vi "iWorx - Force.vi"() -> ()   [LabVIEW 2012]
uses:
  <vilib>/DAQmx/create/channels.llb/DAQmx Create Channel (AI-Voltage-Basic).vi
  <vilib>/DAQmx/read.llb/DAQmx Read (Analog 1D Wfm NChan 1Samp).vi
  <vilib>/ptbypt/NI_PtbyPt.lvlib
panel:
  in  "Set Up":bool
  out "Offset":dbl=-0.0016949152542372892
  out "Slope":dbl=0.33898305084745767
  in  "Set SP2":bool
  in  "Set SP1":bool
  in  "Channel":u16(ring) items=["Channel 1", "Channel 2"]
  in  "Calibration Data":T1={"SP1 Voltage"=0.3, "SP2 Voltage"=0.005, "SP1 Value"=0.1, "SP2 Value"=0.0} {"SP2 Value" format="%_3f Kg"; "SP1 Value" format="%_3f Kg"; "SP2 Voltage" format="%.3f V"; "SP1 Voltage" format="%.3f V"}
  in  "Pause Button":bool
  in  "Snapshot":bool
  out "Processed Signal":dbl(knob) caption="Force (Kg)" scale=-5.0..5.0
  in  "stop":bool
  out "Waveform Chart":dbl(graph)
  in  "Sample Timing":u16(ring)=50 items=["20Hz"=50, "5 Hz"=200, "2 Hz"=500, "1 Hz"=1000, ".5 Hz"=2000, ".2 Hz"=5000]
  in  "Clear Chart":bool
  in  "Open Log":bool
  in  "Autoscale Y":bool
  out "Raw Signal":dbl(knob) scale=-2.5..2.5
  # "iWorx - Force - Data Logger"
  # "Sensor Input"
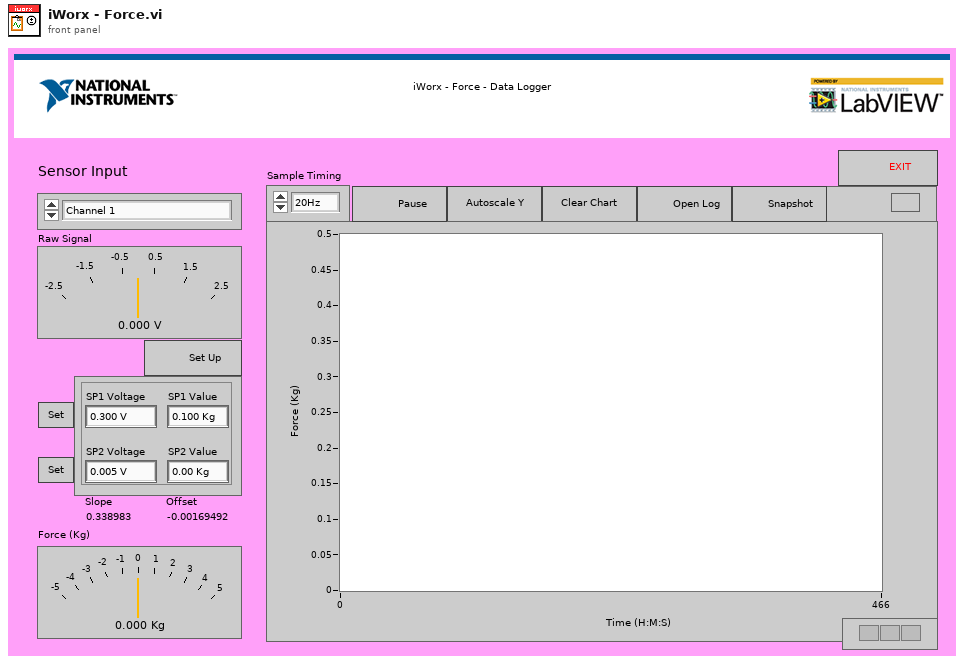
[diagram p1: front panel]
types:
  T1 = cluster{"SP1 Voltage":dbl, "SP2 Voltage":dbl, "SP1 Value":dbl, "SP2 Value":dbl}
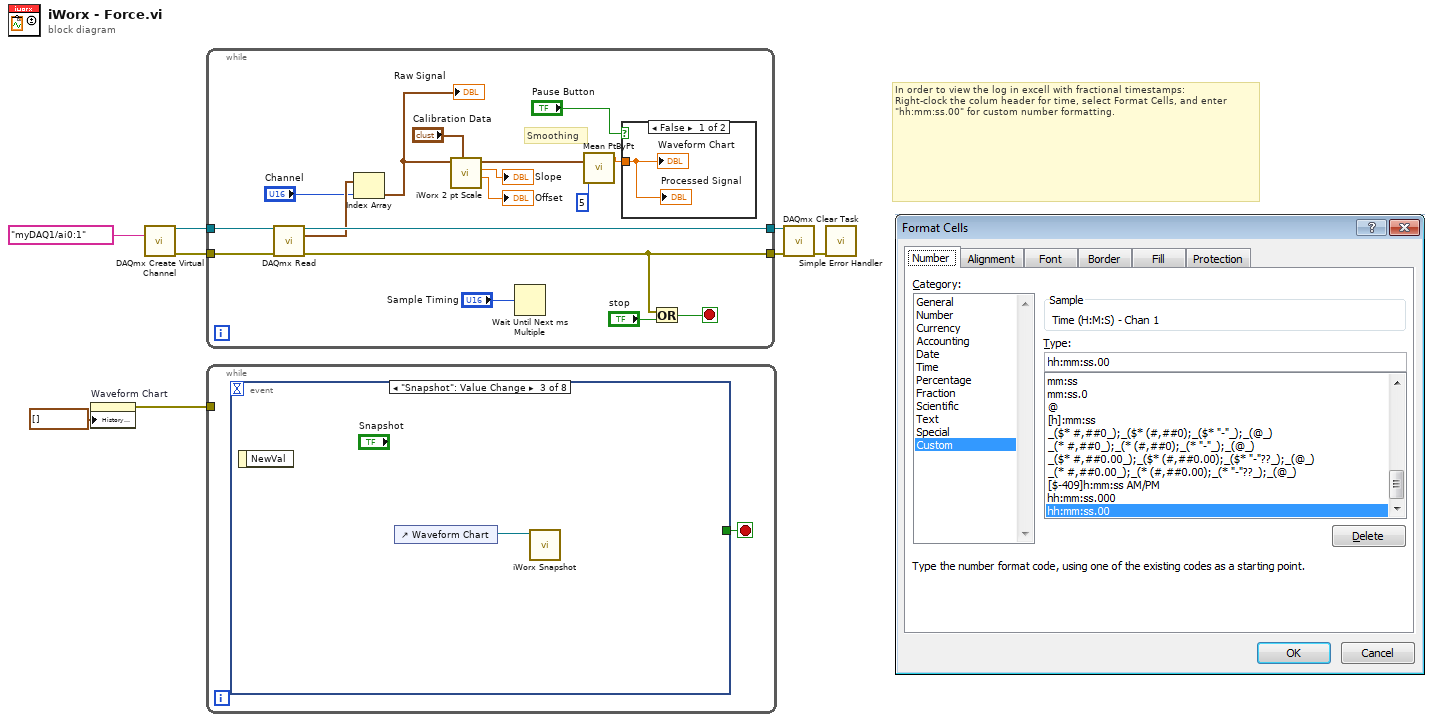
[diagram p0: block diagram]
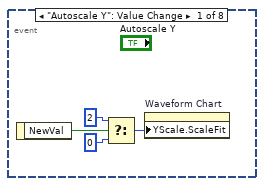
[diagram p2: hidden frame]
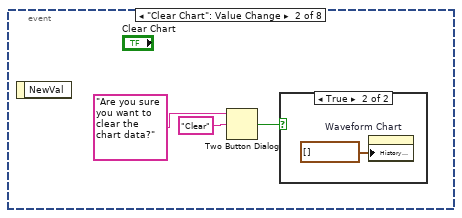
[diagram p3: hidden frame]
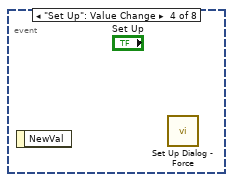
[diagram p5: hidden frame]
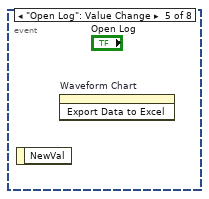
[diagram p6: hidden frame]
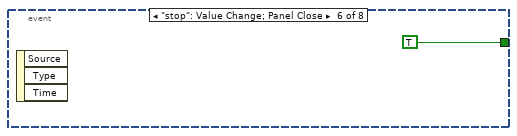
[diagram p7: hidden frame]
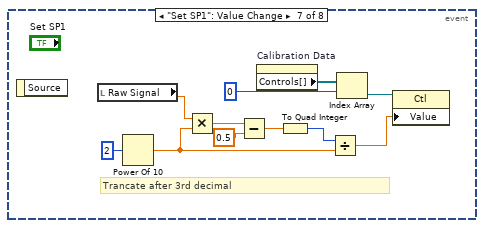
[diagram p8: hidden frame]
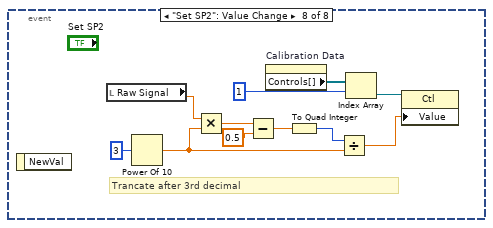
[diagram p9: hidden frame]
diagram:
  # "In order to view the log in excell with fractional timestamps: \nRight-clock the colum header for time, select Format Cells, and enter \"hh:mm:ss.00\" for custom number formatting."
  n1 = property on="Waveform Chart" class="WFChart (strict)"("History Data"=waveform(dbl)[] []) -> (error out=w3:errorcluster)  [unwired: 2 in, 1 out]
  n2 = call-poly <vilib>:"DAQmx Create Virtual Channel.vi"("physical channels"=tag "myDAQ1/ai0:1") -> ("task out"=w5:refnum<k21>, "error out"=w4:errorcluster)  [unwired: 13 in]
  n3 = while {
    tunnel: w5 -> [w23]
    tunnel: [w22] -> w8
    tunnel: w4 -> [w21]
    tunnel: [w19] -> w7
    stop <- w20 stop-if-true
    # "Smoothing"
    n4 = call-poly <vilib>:"DAQmx Read.vi"("task/channels in"=w23, "error in"=w21) -> ("task out"=w22:refnum<k21>, "data"=w17:waveform(dbl)[], "error out"=w19:errorcluster)  [unwired: 11 in]
    n5 = Index Array(array=w17, index="Channel") -> (element=w12:waveform(dbl))
    "Raw Signal" <- w12
    n6 = call "iWorx 2 pt Scale.vi"("Set Points"="Calibration Data", "Raw Waveform"=w12) -> ("Offset"=→"Offset":dbl, "Slope"=→"Slope":dbl, "Scaled Value"=w11:waveform(dbl))  [unwired: 7 in]
    n7 = Wait Until Next ms Multiple(millisecond multiple="Sample Timing") -> ()  [unwired: 1 out]
    n8 = call <vilib>:"Mean PtByPt.vi"("x"=w11, "sample length"=5) -> ("mean"=w10:dbl)  [unwired: 2 in, 1 out]
    n9 = case shown="False" "Pause Button" {
      tunnel: w10 -> [w26 _]
      frame False {
        "Waveform Chart" <- w26
        "Processed Signal" <- w26
      }
      frame True {
      }
    }
    n10 = Or(x=w19, y="stop") -> (x .or. y?=w20:bool)
  }
  n11 = while {
    tunnel: w3 -> [_]
    stop <- w27 stop-if-true
    n12 = event shown="[2] \"Snapshot\": Value Change" {
      selector: _ -> [_ _ _ _ _ _ _ _]
      dyn-events: _ -> [_ _ _ _ _ _ _ _]
      timeout: _ -> [_ _ _ _ _ _ _ _]
      tunnel: [_ _ _ _ _ TRUE _ _] -> w27
      event "Autoscale Y": Value Change {
        n13 = event-data() -> ("NewVal"=w29:bool)  [unwired: 1 in]
        n14 = Select(t=u8 2 ("Y Scale.Scale Fit"), s=w29, f=u8 0 ("Y Scale.Scale Fit")) -> (s? t:f=w28:u8)
        n15 = property on="Waveform Chart" class="WFChart (strict)"("YScale.ScaleFit"=w28) -> ()  [unwired: 2 in, 2 out]
      }
      event "Clear Chart": Value Change {
        n16 = event-data() -> ()  [unwired: 1 in, 1 out]
        n17 = Two Button Dialog(message="Are you sure you want to clear the chart data?", 2:"Clear" ("T button name (\"OK\")")) -> (T button?=w33:bool)  [unwired: 1 in]
        n18 = case shown="True" w33 {
          frame False {
          }
          frame True {
            n19 = property on="Waveform Chart" class="WFChart (strict)"("History Data"=waveform(dbl)[] []) -> ()  [unwired: 2 in, 2 out]
          }
        }
      }
      event "Snapshot": Value Change {
        n20 = event-data() -> ()  [unwired: 1 in, 1 out]
        n21 = control-ref of="Waveform Chart"() -> (w36:refnum<vi>)
        n22 = call "iWorx Snapshot.vi"("WaveformChart in"=w36) -> ()  [unwired: 10 in, 1 out]
      }
      event "Set Up": Value Change {
        n23 = event-data() -> ()  [unwired: 1 in, 1 out]
        n24 = call "Set Up Dialog - Force.vi"() -> ()  [unwired: 12 in]
      }
      event "Open Log": Value Change {
        n25 = event-data() -> ()  [unwired: 1 in, 1 out]
        n26 = invoke on="Waveform Chart" class="WFChart (strict)" method="Export Data to Excel"() -> ()  [unwired: 3 in, 3 out]
      }
      event "stop": Value Change; Panel Close {
        n27 = event-data() -> ()  [unwired: 1 in, 3 out]
      }
      event "Set SP1": Value Change {
        # "Trancate after 3rd decimal"
        n28 = event-data() -> ()  [unwired: 1 in, 1 out]
        n29 = local read "Raw Signal"() -> (w38:dbl)
        n30 = Power Of 10(x=2) -> (10^x=w45:dbl)
        n31 = Multiply(x=w38, y=w45) -> (x*y=w43:dbl)
        n32 = Subtract(x=w43, y=0.5) -> (x-y=w42:dbl)
        n33 = property on="Calibration Data" class="Clust (strict)"() -> ("Controls[]"=w48:refnum<vi>[])  [unwired: 2 in, 2 out]
        n34 = To Quad Integer(1:w42) -> (0:w44:i64)
        n35 = Divide(x=w44, y=w45) -> (x/y=w40:dbl)
        n36 = Index Array(array=w48, index=0) -> (element=w47:refnum<vi>)
        n37 = property class="Ctl"(reference=w47, "Value"=w40) -> ()  [unwired: 1 in, 2 out]
      }
      event "Set SP2": Value Change {
        # "Trancate after 3rd decimal"
        n38 = event-data() -> ()  [unwired: 1 in, 1 out]
        n39 = local read "Raw Signal"() -> (w49:dbl)
        n40 = Power Of 10(x=3) -> (10^x=w56:dbl)
        n41 = Multiply(x=w49, y=w56) -> (x*y=w54:dbl)
        n42 = Subtract(x=w54, y=0.5) -> (x-y=w53:dbl)
        n43 = property on="Calibration Data" class="Clust (strict)"() -> ("Controls[]"=w59:refnum<vi>[])  [unwired: 2 in, 2 out]
        n44 = To Quad Integer(1:w53) -> (0:w55:i64)
        n45 = Divide(x=w55, y=w56) -> (x/y=w51:dbl)
        n46 = Index Array(array=w59, index=1) -> (element=w58:refnum<vi>)
        n47 = property class="Ctl"(reference=w58, "Value"=w51) -> ()  [unwired: 1 in, 2 out]
      }
    }
  }
  n48 = call <vilib>:"DAQmx Clear Task.vi"("task in"=w8, "error in"=w7) -> ("error out"=w2:errorcluster)  [unwired: 13 in]
  n49 = call <vilib>:"Simple Error Handler.vi"("error in (no error)"=w2) -> ()  [unwired: 4 in, 5 out]
